vi "store2ADCToFileHeader.vi"(0 "chipNumber":string, 1 "MuxChan":i32, 2 "minAttenuator":i32=127, 3 "maxAttenuator":i32=127, 4 "totalRepetitionsToDo":u32, 5 "ADCselect":enum16{"ADC18", "ADC16", "2ADC", "None"}(ring)=enum."2ADC", 7 "aspic2Data 2":u32[](array[numeric])=[170, 187, 204, 221, 238, 255, 10, 10, 10, 10, 10, 10, 10, 10, 10, 10, 10, 10, 10, 10, 10, 10, 10, 10, 10, 10, 10, 10, 10, 10, 10, 10] format="%07x", 9 "Write to disk":T1(ring), 11 "Test type":T2(ring), 12 "current time":timestamp, 13 "comments":string, 14 "inputVoltage":dbl) -> (15 "error out":errorcluster)   [LabVIEW 2014]
uses:
  Global 1.vi
panel:
  out "typeTest":string
  out "justTime":string
  out "justDate":string
  out "outputFileName":string
  out "datetime":string
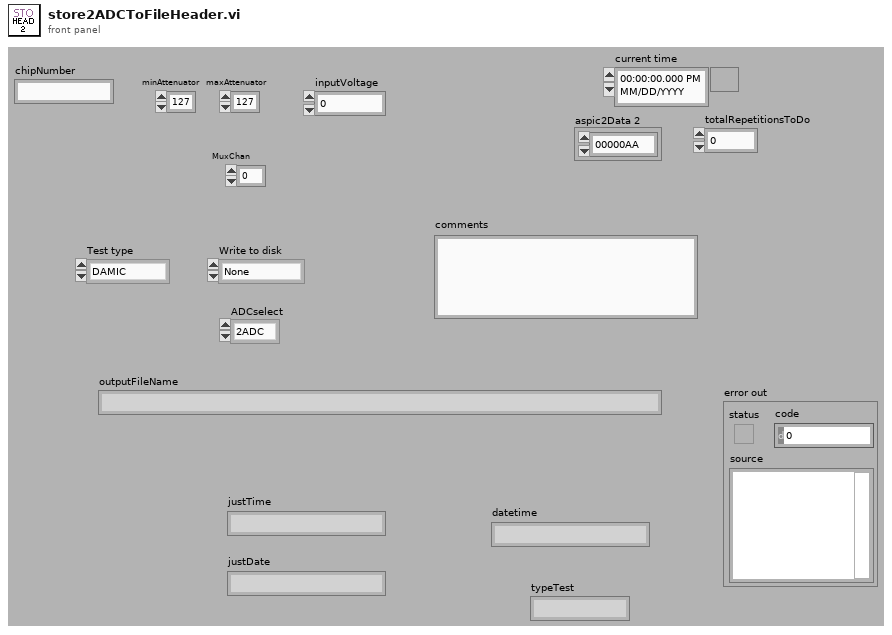
[diagram p1: front panel]
types:
  T1 = enum16{"None", "Average", "StdDev", "AvgStdDev", "ChanAverage", "All"}
  T2 = enum16{"DAMIC", "NOISE", "GAIN", "LINEAR18", "XTALK", "TEMP", "LINEAR16", "CONSO"}
  T3 = enum16{"open", "replace", "create", "open or create", "replace or create", "replace or create with confirmation"}
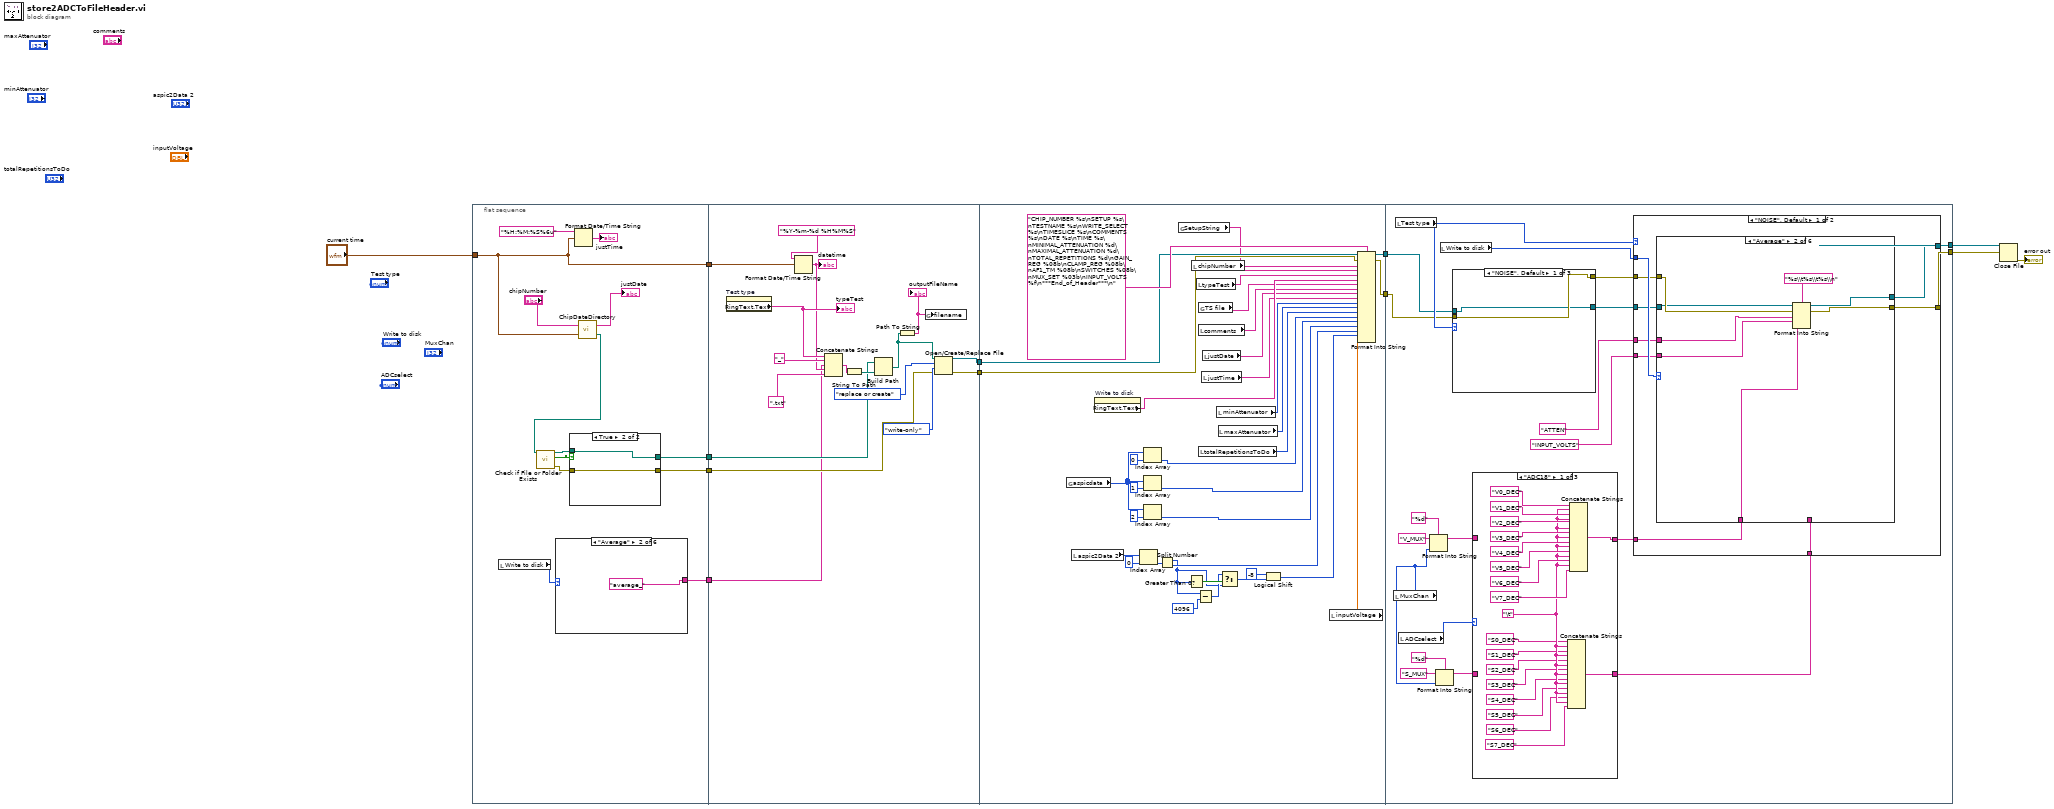
[diagram p0: block diagram]
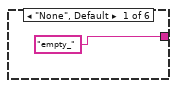
[diagram p2: hidden frame]
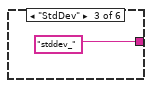
[diagram p3: hidden frame]
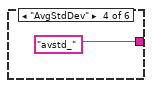
[diagram p4: hidden frame]
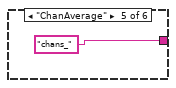
[diagram p5: hidden frame]
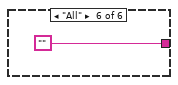
[diagram p6: hidden frame]
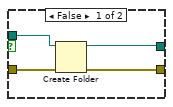
[diagram p7: hidden frame]
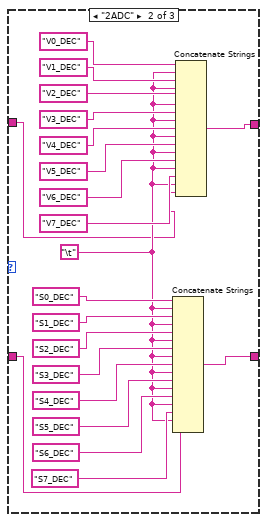
[diagram p8: hidden frame]
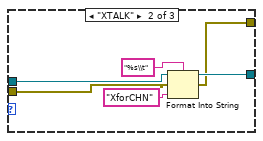
[diagram p10: hidden frame]
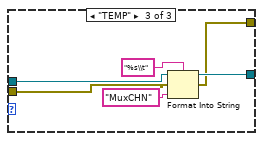
[diagram p11: hidden frame]
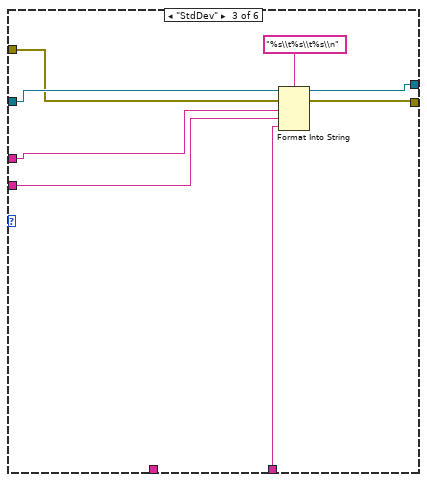
[diagram p13: hidden frame]
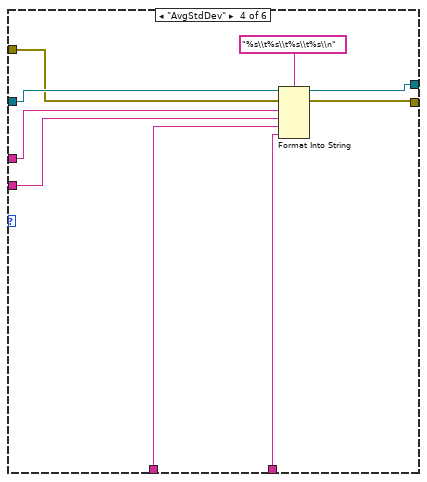
[diagram p14: hidden frame]
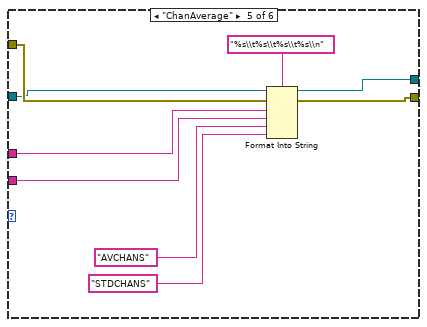
[diagram p15: hidden frame]
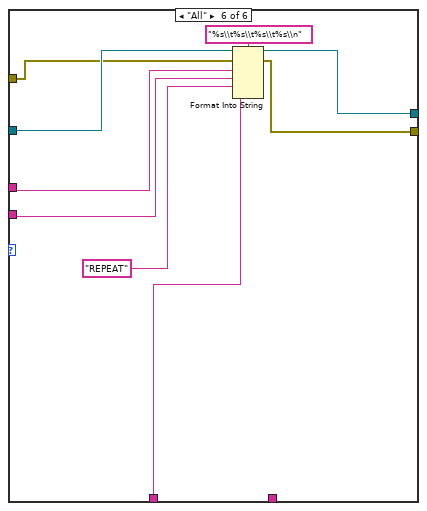
[diagram p16: hidden frame]
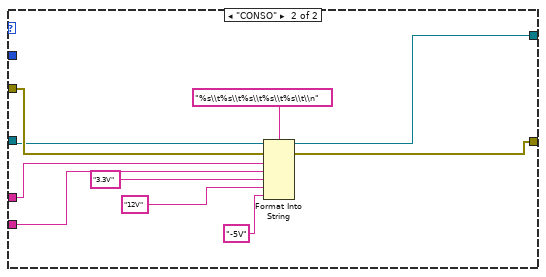
[diagram p17: hidden frame]
diagram:
  n1 = flat-sequence {
    tunnel: "current time" -> [w16]
    tunnel: [w16] -> w5
    tunnel: [w22] -> w4
    tunnel: [w19] -> w3
    tunnel: [w17] -> w2
    tunnel: [w51] -> w7
    tunnel: [w50] -> w6
    tunnel: w5 -> [w48]
    tunnel: w4 -> [w44]
    tunnel: w3 -> [w43]
    tunnel: w2 -> [w38]
    tunnel: [w89] -> w8
    tunnel: [w88] -> w9
    tunnel: w7 -> [w77]
    tunnel: w6 -> [w76]
    tunnel: [w108] -> w11
    tunnel: [w109] -> w12
    tunnel: w9 -> [w105]
    tunnel: w8 -> [w106]
    frame #0 {
      n2 = local read "Write to disk"() -> (w18:T1)
      n3 = case shown="\"Average\"" w18 {
        tunnel: ["empty_" "average_" "stddev_" "avstd_" "chans_" ""] -> w17
        frame "None", Default {
        }
        frame "Average" {
        }
        frame "StdDev" {
        }
        frame "AvgStdDev" {
        }
        frame "ChanAverage" {
        }
        frame "All" {
        }
      }
      n4 = Format Date/Time String(time format string (%c)="%H:%M:%S%6u", seconds (now)=w16) -> (date/time string=→"justTime":string)  [unwired: 1 in]
      n5 = call "ChipDateDirectory.vi"("time stamp"=w16, "chipNumber"="chipNumber") -> ("path"=w13:path, "justDate"=→"justDate":string)
      n6 = call <vilib>:"Check if File or Folder Exists.vi"("path"=w13) -> ("error out"=w20:errorcluster, "file or folder exists?"=w23:bool, "dup path"=w21:path)  [unwired: 1 in, 7 out]
      n7 = case shown="True" w23 {
        tunnel: [w34 w37] -> w22
        tunnel: w21 -> [w35 w37]
        tunnel: w20 -> [w33 w36]
        tunnel: [w32 w36] -> w19
        frame False {
          n8 = Create Folder(path (use dialog)=w35, error in=w33) -> (created path=w34:path, error out=w32:errorcluster)  [unwired: 2 out]
        }
        frame True {
        }
      }
    }
    frame #1 {
      n9 = property on="Test type" class="Enum (strict)"() -> ("RingText.Text"=w47:string)  [unwired: 2 in, 2 out]
      "typeTest" <- w47
      n10 = Format Date/Time String(time format string (%c)="%Y-%m-%d %H%M%S", seconds (now)=w48) -> (date/time string=w39:string)  [unwired: 1 in]
      "datetime" <- w39
      n11 = Concatenate Strings(w47, "_", w38, w39, ".txt" ("string")) -> (w54:string)
      n12 = String To Path(string=w54) -> (path=w46:path)
      n13 = Build Path(base path=w44, name or relative path=w46) -> (appended path=w45:path)
      n14 = Path To String(path=w45) -> (string=w42:string)
      "outputFileName" <- w42
      n15 = global write "Global 1.vi" "filename"(w42) -> ()
      n16 = Open/Create/Replace File(file path (use dialog)=w45, error in=w43, operation (0:open)=T3."replace or create", access (0:read/write)=enum16{"read/write", "read-only", "write-only"}."write-only") -> (refnum out=w51:refnum<file>, error out=w50:errorcluster)  [unwired: 3 out]
    }
    frame #2 {
      n17 = global read "Global 1.vi" "aspicdata"() -> (w57:u32[])
      n18 = local read "aspic2Data 2"() -> (w85:u32[])
      n19 = property on="Write to disk" class="Enum (strict)"() -> ("RingText.Text"=w74:string)  [unwired: 2 in, 2 out]
      n20 = Index Array(array=w85, index=0) -> (element=w78:u32)
      n21 = Index Array(array=w57, index=0) -> (element=w60:u32)
      n22 = Index Array(array=w57, index=1) -> (element=w59:u32)
      n23 = Index Array(array=w57, index=2) -> (element=w58:u32)
      n24 = Split Number(x=w78) -> (hi(x)=w64:u16, lo(x)=w65:u16)
      n25 = global read "Global 1.vi" "SetupString"() -> (w55:string)
      n26 = Greater Than 0?(x=w64) -> (x > 0?=w67:bool)
      n27 = local read "chipNumber"() -> (w81:string)
      n28 = local read "typeTest"() -> (w56:string)
      n29 = Subtract(x=w64, y=u16 4096) -> (x-y=w66:u16)
      n30 = local read "comments"() -> (w72:string)
      n31 = local read "totalRepetitionsToDo"() -> (w79:u32)
      n32 = global read "Global 1.vi" "TS file"() -> (w73:string)
      n33 = local read "justTime"() -> (w71:string)
      n34 = local read "justDate"() -> (w70:string)
      n35 = local read "minAttenuator"() -> (w75:i32)
      n36 = local read "maxAttenuator"() -> (w80:i32)
      n37 = Select(t=w66, s=w67, f=w64) -> (s? t:f=w63:u16)
      n38 = Logical Shift(y=i8 -8, x=w63) -> (x << y=w62:u16)
      n39 = local read "inputVoltage"() -> (w68:dbl)
      n40 = Format Into String(format string="CHIP_NUMBER %s\nSETUP %s\nTESTNAME %s\nWRITE_SELECT %s\nTIMESLICE %s\nCOMMENTS %s\nDATE %s\nTIME %s\nMINIMAL_ATTENUATION %d\nMAXIMAL_ATTENUATION %d\nTOTAL_REPETITIONS %d\nGAIN_REG %08b\nCLAMP_REG %08b\nAF1_TM %08b\nSWITCHES %08b\nMUX_SET %03b\nINPUT_VOLTS %f\n***End_of_Header***\n", initial string=w77, error in=w76, w81, w55, w56, w74, w73, w72, w70, w71, w75, w80, w79, w60, w59, w58, w65, w62, w68) -> (resulting string=w89:refnum<file>, error out=w88:errorcluster)
    }
    frame #3 {
      n41 = local read "MuxChan"() -> (w91:i32)
      n42 = local read "Test type"() -> (w107:T2)
      n43 = local read "ADCselect"() -> (w97:enum16{"ADC18", "ADC16", "2ADC", "None"})
      n44 = Format Into String(format string="%d", initial string="V_MUX" ("input 2"), w91) -> (resulting string=w95:string)  [unwired: 1 in, 1 out]
      n45 = Format Into String(format string="%d", initial string="S_MUX" ("input 2"), w91) -> (resulting string=w90:string)  [unwired: 1 in, 1 out]
      n46 = local read "Write to disk"() -> (w102:T1)
      n47 = case shown="\"NOISE\", Default" w107 {
        tunnel: w106 -> [w152 w157 w163]
        tunnel: w105 -> [w153 w156 w162]
        tunnel: [w152 w155 w161] -> w104
        tunnel: [w153 w154 w160] -> w103
        frame "NOISE", Default {
        }
        frame "XTALK" {
          n48 = Format Into String(format string="%s\\t", initial string=w157, error in=w156, "XforCHN" ("input 11")) -> (resulting string=w155:refnum<file>, error out=w154:errorcluster)
        }
        frame "TEMP" {
          n49 = Format Into String(format string="%s\\t", initial string=w163, error in=w162, "MuxCHN" ("input 11")) -> (resulting string=w161:refnum<file>, error out=w160:errorcluster)
        }
      }
      n50 = case shown="\"ADC18\"" w97 {
        tunnel: [w120 w141 w151] -> w99
        tunnel: [w110 w132 w150] -> w98
        tunnel: w95 -> [_ w130 w151]
        tunnel: w90 -> [_ w129 w150]
        frame "ADC18" {
          w119 = "\t"
          n51 = Concatenate Strings("S0_DEC" ("input 2"), w119, "S1_DEC" ("input 2"), w119, "S2_DEC" ("input 2"), w119, "S3_DEC" ("input 2"), w119, "S4_DEC" ("input 2"), w119, "S5_DEC" ("input 2"), w119, "S6_DEC" ("input 2"), w119, "S7_DEC" ("input 2")) -> (w110:string)
          n52 = Concatenate Strings("V0_DEC" ("input 2"), w119, "V1_DEC" ("input 2"), w119, "V2_DEC" ("input 2"), w119, "V3_DEC" ("input 2"), w119, "V4_DEC" ("input 2"), w119, "V5_DEC" ("input 2"), w119, "V6_DEC" ("input 2"), w119, "V7_DEC" ("input 2")) -> (w120:string)
        }
        frame "2ADC" {
          w131 = "\t"
          n53 = Concatenate Strings("S0_DEC" ("input 2"), w131, "S1_DEC" ("input 2"), w131, "S2_DEC" ("input 2"), w131, "S3_DEC" ("input 2"), w131, "S4_DEC" ("input 2"), w131, "S5_DEC" ("input 2"), w131, "S6_DEC" ("input 2"), w131, "S7_DEC" ("input 2"), w131, w129) -> (w132:string)
          n54 = Concatenate Strings("V0_DEC" ("input 2"), w131, "V1_DEC" ("input 2"), w131, "V2_DEC" ("input 2"), w131, "V3_DEC" ("input 2"), w131, "V4_DEC" ("input 2"), w131, "V5_DEC" ("input 2"), w131, "V6_DEC" ("input 2"), w131, "V7_DEC" ("input 2"), w131, w130) -> (w141:string)
        }
        frame "ADC16", Default {
        }
      }
      n55 = case shown="\"NOISE\", Default" w107 {
        tunnel: [w170 w226] -> w109
        tunnel: [w174 w225] -> w108
        tunnel: w104 -> [w171 w227]
        tunnel: w103 -> [w172 w228]
        tunnel: w102 -> [w173 _]
        tunnel: "ATTEN" ("input 11") -> [w169 w224]
        tunnel: "INPUT_VOLTS" ("input 11") -> [w168 w223]
        tunnel: w99 -> [w167 _]
        tunnel: w98 -> [w166 _]
        frame "NOISE", Default {
          n56 = case shown="\"Average\"" w173 {
            tunnel: [w175 w183 w191 w200 w205 w218] -> w170
            tunnel: [w176 w182 w190 w199 w204 w217] -> w174
            tunnel: w172 -> [w176 w181 w188 w197 w207 w214]
            tunnel: w171 -> [w175 w180 w189 w198 w206 w215]
            tunnel: w169 -> [_ w179 w187 w196 w203 w213]
            tunnel: w168 -> [_ w178 w186 w195 w202 w212]
            tunnel: w167 -> [_ w177 _ w194 _ w211]
            tunnel: w166 -> [_ _ w185 w193 _ _]
            frame "None", Default {
            }
            frame "Average" {
              n57 = Format Into String(format string="%s\\t%s\\t%s\\n", initial string=w180, error in=w181, w179, w178, w177) -> (resulting string=w183:refnum<file>, error out=w182:errorcluster)
            }
            frame "StdDev" {
              n58 = Format Into String(format string="%s\\t%s\\t%s\\n", initial string=w189, error in=w188, w187, w186, w185) -> (resulting string=w191:refnum<file>, error out=w190:errorcluster)
            }
            frame "AvgStdDev" {
              n59 = Format Into String(format string="%s\\t%s\\t%s\\t%s\\n", initial string=w198, error in=w197, w196, w195, w194, w193) -> (resulting string=w200:refnum<file>, error out=w199:errorcluster)
            }
            frame "ChanAverage" {
              n60 = Format Into String(format string="%s\\t%s\\t%s\\t%s\\n", initial string=w206, error in=w207, w203, w202, "AVCHANS" ("input 2"), "STDCHANS" ("input 2")) -> (resulting string=w205:refnum<file>, error out=w204:errorcluster)
            }
            frame "All" {
              n61 = Format Into String(format string="%s\\t%s\\t%s\\t%s\\n", initial string=w215, error in=w214, w213, w212, "REPEAT" ("input 11"), w211) -> (resulting string=w218:refnum<file>, error out=w217:errorcluster)
            }
          }
        }
        frame "CONSO" {
          n62 = Format Into String(format string="%s\\t%s\\t%s\\t%s\\t%s\\t\\n", initial string=w227, error in=w228, w224, w223, "3.3V" ("input 3"), "12V" ("input 4"), "-5V" ("input 5")) -> (resulting string=w226:refnum<file>, error out=w225:errorcluster)
        }
      }
    }
  }
  n63 = Close File(refnum=w12, error in=w11) -> (error out=→"error out":errorcluster)  [unwired: 1 out]
